vi "Initialize and Configure.vi"(6 "trigger mode (0:internal)":u16(ring) items=["internal - continuous trigger", "external - rear panel trigger with delay", "external - bus trigger with delay", "external - rear panel trigger", "external - bus trigger"], 7 "function (0:volts DC)":u16(ring) items=["volts DC", "volts AC", "2-wire k.ohms", "4-wire k.ohms", "mA DC", "mA AC"], 8 "error in (no error)":errorcluster, 9 "rate (0:slow)":u16(ring) items=["slow", "medium", "fast"], 10 "range (0:auto)":u16(ring) items=["autorange", "200mV, 200 ohms", "2V, 2 kohms", "20V, 20 kohms", "200V, 200 kohms", "1000Vdc, 700 Vac, 2 Mohms", "20 Mohms", "20 mV, 20 ohms"], 11 "Fluke Multimeter.lvclass In":refnum<class "Fluke Multimeter.lvclass">) -> (0 "error out":errorcluster, 3 "Fluke Multimeter.lvclass Out":refnum<class "Fluke Multimeter.lvclass">)   [LabVIEW 2023, in "Fluke Multimeter.lvclass"]
doc: "Initializes and configures the Fluke Multimeter."
uses:
  Fluke Multimeter.lvclass
  Fluke Multimeter.lvclass/Fluke Multimeter.ctl
  Fluke 8840/Fluke 8840.lvlib
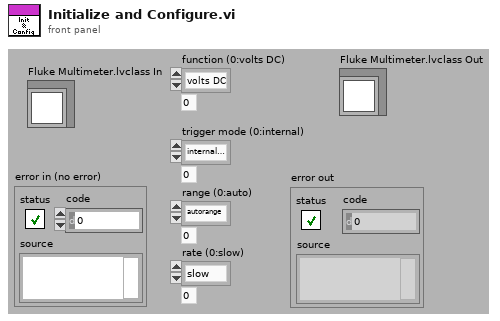
[diagram p1: front panel]
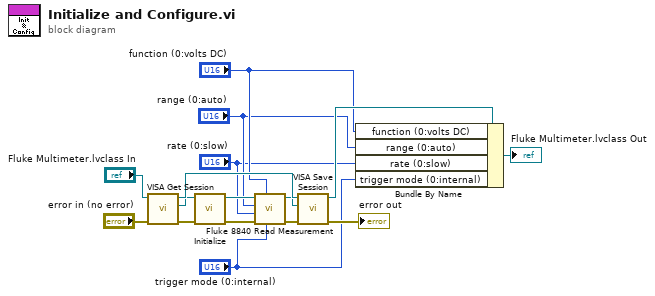
[diagram p0: block diagram]
diagram:
  n1 = call-dynamic "VISA Get Session.vi"("error in (no error)"="error in (no error)", "Instrument.lvclass in"="Fluke Multimeter.lvclass In") -> ("error out"=w11:errorcluster, "VISA Resource Name"=w12:refnum<visa-resource-name>, "Instrument.lvclass out"=w13:refnum<class "Fluke Multimeter.lvclass">)  [unwired: 7 out]
  n2 = call "Initialize.vi"("error in (no error)"=w11, "VISA resource name"=w12) -> ("error out"=w9:errorcluster, "VISA resource name out"=w10:refnum<visa-resource-name>)  [unwired: 8 in]
  n3 = call "Fluke 8840 Read Measurement.vi"("trigger mode (0:internal)"="trigger mode (0:internal)", "function (0:volts DC)"="function (0:volts DC)", "error in (no error)"=w9, "rate (0:slow)"="rate (0:slow)", "range (0:auto)"="range (0:auto)", "VISA resource name"=w10) -> ("error out"=w7:errorcluster, "VISA resource name out"=w8:refnum<visa-resource-name>)  [unwired: 2 in, 2 out]
  n4 = call-dynamic "VISA Save Session.vi"("error in (no error)"=w7, "VISA Resource Name"=w8, "Instrument.lvclass in"=w13) -> ("error out"=→"error out":errorcluster, "Instrument.lvclass out"=w6:refnum<class "Fluke Multimeter.lvclass">)  [unwired: 7 out]
  n5 = Bundle By Name(cluster=w6, "function (0:volts DC)"="function (0:volts DC)", "range (0:auto)"="range (0:auto)", "rate (0:slow)"="rate (0:slow)", "trigger mode (0:internal)"="trigger mode (0:internal)") -> (→"Fluke Multimeter.lvclass Out":refnum<class "Fluke Multimeter.lvclass">)
